vi "Constructor.vi"(7 "Frequency":dbl, 8 "error in (no error)":errorcluster, 9 "Negative Pole":i32, 10 "Positive Pole":i32, 11 "VISA resource name":refnum<visa-resource-name>) -> (0 "error out":errorcluster, 3 "Motor out":refnum<class "Motor.lvclass">)   [LabVIEW 2026, in "Motor.lvlib" / "Motor.lvclass"]
uses:
  Motor.lvclass
  Motor.lvclass/Motor.ctl
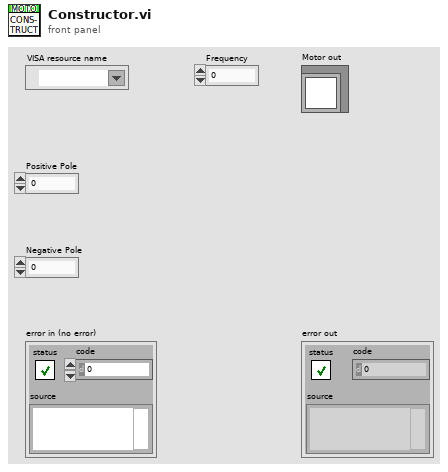
[diagram p1: front panel]
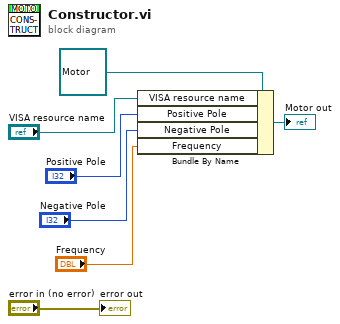
[diagram p0: block diagram]
diagram:
  n1 = Bundle By Name(cluster=refnum<class "Motor.lvclass"> refnum ("Motor in"), "VISA resource name"="VISA resource name", "Positive Pole"="Positive Pole", "Negative Pole"="Negative Pole", "Frequency"="Frequency") -> (→"Motor out":refnum<class "Motor.lvclass">)
  "error out" <- "error in (no error)"
